vi "Søg hel string float32.vi"() -> ()   [LabVIEW 2018]
uses:
  <vilib>/Utility/file.llb/Write Delimited Spreadsheet (DBL).vi
panel:
  out "appended array":dbl[](array[numeric])
  out "substring":string
  in  "String input":string="–¼ ×¤<Ã}"
  out "I_Longi direkte grader":dbl
  out "I_Latti direkte grader":dbl
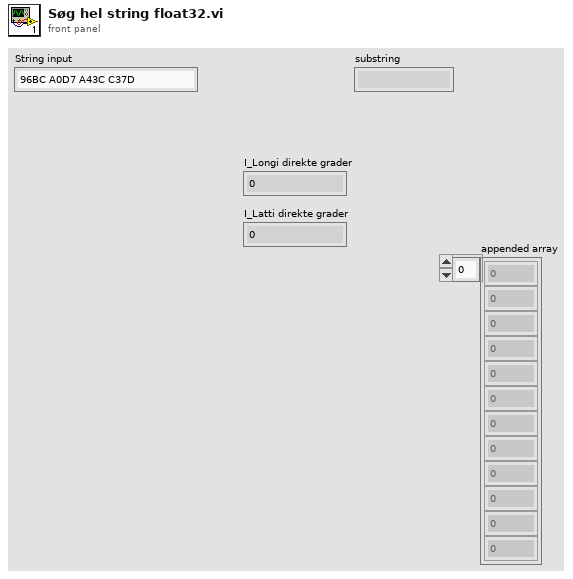
[diagram p1: front panel]
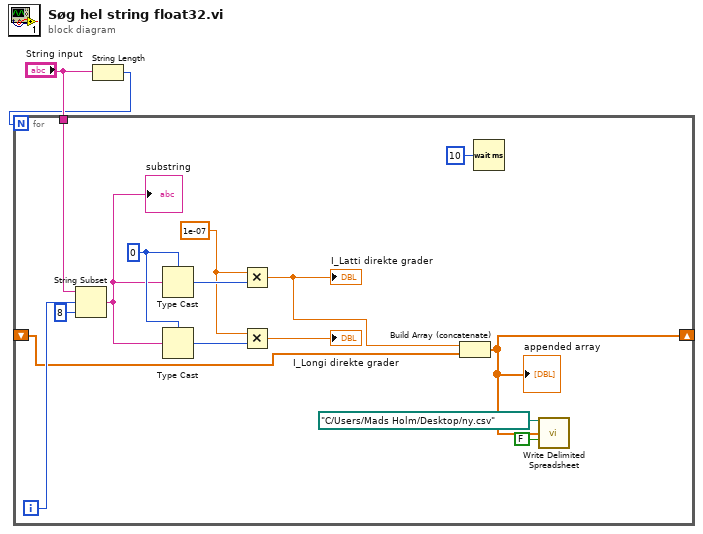
[diagram p0: block diagram]
diagram:
  n1 = String Length(string="String input") -> (length=w1:i32)
  n2 = for {
    N: w1 -> [_]
    tunnel: "String input" -> [w10]
    shift-right: [w5] -> _
    shift-left: _ -> [w6]
    i -> [w12]
    w13 = 1e-07 ("y")
    w17 = 0
    n3 = String Subset(string=w10, offset (0)=w12, length (rest)=8 ("length (rest)")) -> (substring=w11:string)
    "substring" <- w11
    n4 = Type Cast(type=w17, x=w11) -> (*(type *) &x=w16:i32)
    n5 = Type Cast(type=w17, x=w11) -> (*(type *) &x=w15:i32)
    n6 = Multiply(x=w13, y=w16) -> (x*y=w7:dbl)
    "I_Latti direkte grader" <- w7
    n7 = Multiply(x=w13, y=w15) -> (x*y=→"I_Longi direkte grader":dbl)
    n8 = Build Array (concatenate)(w7, w6) -> (w5:dbl[])
    "appended array" <- w5
    n9 = Wait (ms)(milliseconds to wait=u32 10) -> ()  [unwired: 1 out]
    n10 = call-poly <vilib>:"Write Delimited Spreadsheet.vi"("file path (dialog if empty)"=path "C:/Users/Mads Holm/Desktop/ny.csv", "1D data"=w5, "append to file? (new file:F)"=FALSE) -> ()  [unwired: 11 in, 2 out]
  }
